vi "Global Resources Mod.vi"(7 "Path to All Nodes Resources":string="IONode\\Controls\\All Nodes Resources.ctl", 8 "error in":errorcluster, 10 "Number of SPI Devices on Bus":i32=1 min=1 step=1, 11 "Path to IO Node":path=path "D:/Documents/Projects/SPIAPI/IOEngineCode/Initialize Node Resources.vi") -> (0 "error out":errorcluster, 2 "Number of SPI Devices on Bus":i32=1 min=1 step=1, 3 "Path to IO Node":path=path "D:/Documents/Projects/SPIAPI/IOEngineCode/Initialize Node Resources.vi")   [LabVIEW 2014, in "Initialization and IO Node Scripting.lvlib"]
uses:
  Initialization and IO Node Scripting.lvlib
  <vilib>/Utility/traverseref.llb/TRef TravTarget.ctl
  <vilib>/Utility/traverseref.llb/VI Scripting - Traverse.lvlib
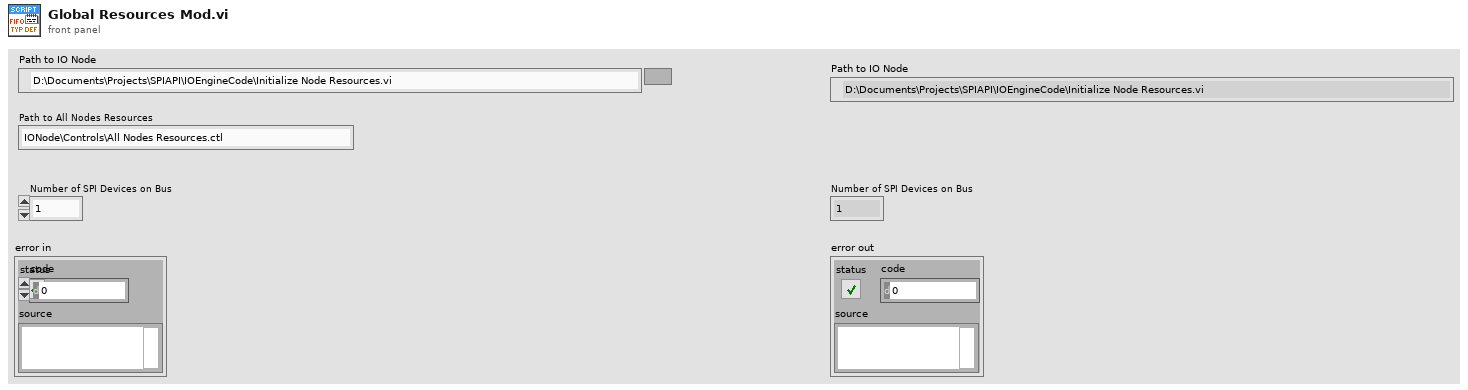
[diagram p1: front panel]
types:
  T1 = typedef "TRef TravTarget.ctl" = enum16{"FP", "BD", "Other"}
  T2 = typedef "LVPositionTypeDef.ctl" = cluster{"Left":i32, "Top":i32}
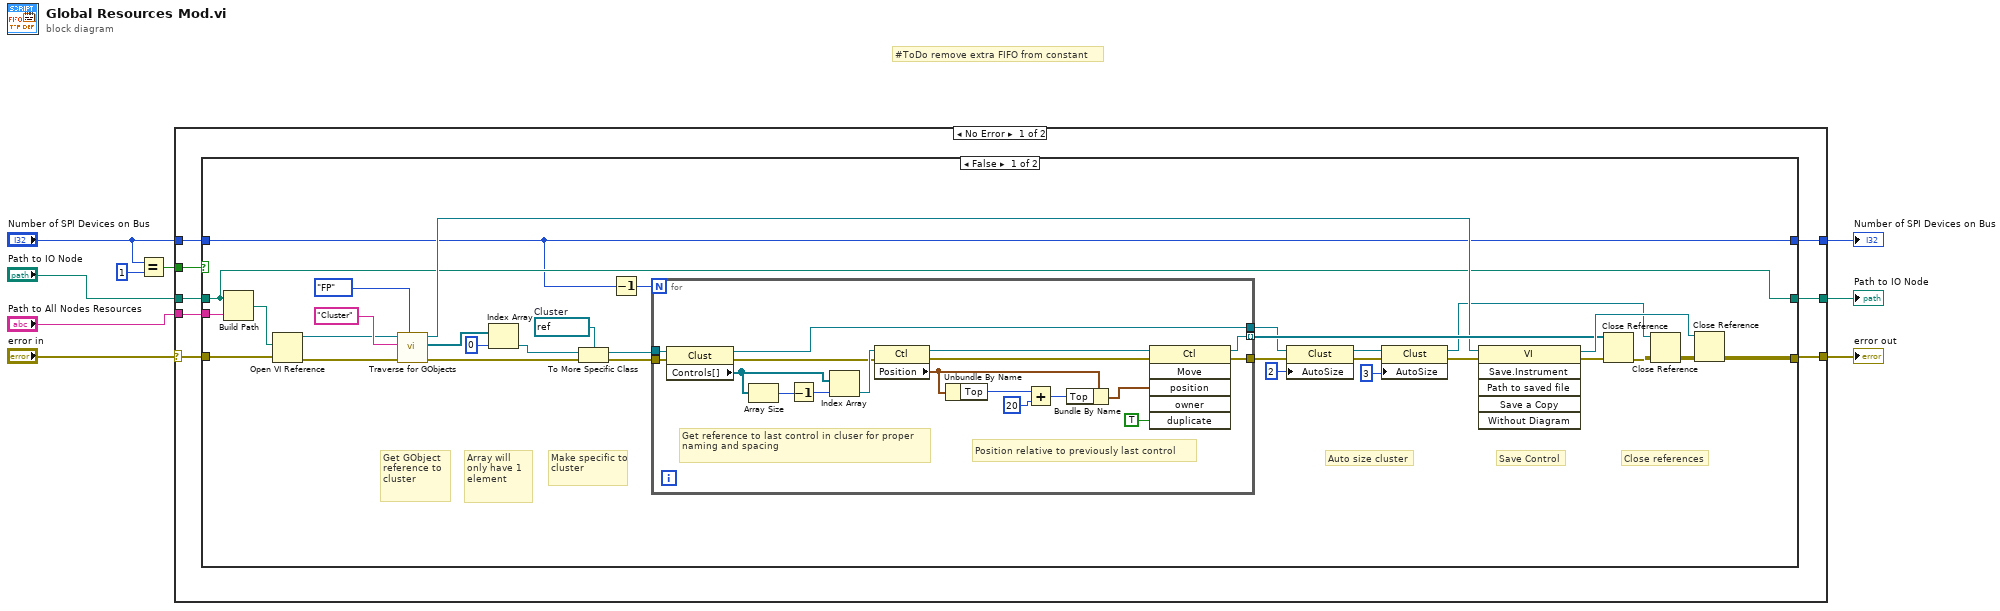
[diagram p0: block diagram]
diagram:
  # "#ToDo remove extra FIFO from constant"
  n1 = Equal?(x="Number of SPI Devices on Bus", y=1) -> (x = y?=w7:bool)
  n2 = case shown="No Error" "error in" {
    selector: "error in" -> [w13 w73]
    tunnel: [w17 w73] -> w9
    tunnel: "Path to IO Node" -> [w16 w71]
    tunnel: w7 -> [w15 _]
    tunnel: "Number of SPI Devices on Bus" -> [w14 w72]
    tunnel: [w11 w72] -> w3
    tunnel: [w12 w71] -> w2
    tunnel: "Path to All Nodes Resources" -> [w10 _]
    frame No Error {
      n3 = case shown="False" w15 {
        tunnel: [w48 w70] -> w17
        tunnel: w13 -> [w47 w70]
        tunnel: w16 -> [w28 w69]
        tunnel: w14 -> [w27 w68]
        tunnel: [w28 w69] -> w12
        tunnel: [w27 w68] -> w11
        tunnel: w10 -> [w26 _]
        frame False {
          w38 = refnum<vi> refnum  # Cluster
          # "Auto size cluster"
          # "Save Control"
          # "Close references"
          # "Array will only have 1 element"
          # "Make specific to cluster"
          # "Get GObject reference to cluster"
          n4 = Build Path(base path=w28, name or relative path=w26) -> (appended path=w46:path)
          n5 = Open VI Reference(vi path=w46, error in (no error)=w47) -> (vi reference=w43:refnum<vi>, error out=w37:errorcluster)  [unwired: 4 in]
          n6 = call <vilib>:"Traverse for GObjects.vi"("Traverse Target"=TRef_TravTarget."FP", "error in (no error)"=w37, "Class Name"="Cluster", "VI Refnum"=w43) -> ("error out"=w36:errorcluster, "References"=w42:refnum<vi>[], "dup VI Refnum"=w33:refnum<vi>)  [unwired: 4 in, 1 out]
          n7 = Index Array(array=w42, index=0) -> (element=w40:refnum<vi>)
          n8 = To More Specific Class(target class=w38, reference=w40, error in=w36) -> (specific class reference=w39:refnum<vi>, error out=w35:errorcluster)
          n9 = Decrement(x=w27) -> (x-1=w31:i32)
          n10 = for {
            N: w31 -> [_]
            tunnel: [w54] -> w20
            tunnel: w39 -> [w53]
            tunnel: w35 -> [w52]
            tunnel: [w51] -> w34 mode=indexing
            tunnel: [w50] -> w25
            # "Position relative to previously last control"
            # "Get reference to last control in cluser for proper naming and spacing"
            n11 = property class="Clust"(reference=w53, error in=w52) -> (reference out=w50:refnum<vi>, error out=w58:errorcluster, "Controls[]"=w57:refnum<vi>[])
            n12 = Array Size(array=w57) -> (size(s)=w67:i32)
            n13 = Decrement(x=w67) -> (x-1=w56:i32)
            n14 = Index Array(array=w57, index=w56) -> (element=w63:refnum<vi>)
            n15 = property class="Ctl"(reference=w63, error in=w58) -> (reference out=w64:refnum<vi>, error out=w65:errorcluster, "Position"=w61:T2)
            n16 = Unbundle By Name(w61) -> ("Top"=w60:i32)
            n17 = Add(x=w60, y=20) -> (x+y=w59:i32)
            n18 = Bundle By Name(cluster=w61, "Top"=w59) -> (w62:T2)
            n19 = invoke class="Ctl" method="Move"(reference=w64, error in=w65, "position"=w62, "duplicate"=TRUE ("Duplicate? (F)")) -> (reference out=w51:refnum<vi>, error out=w54:errorcluster)  [unwired: 2 in, 4 out]
          }
          n20 = property class="Clust"(reference=w25, error in=w20, "AutoSize"=u32 2 ("Auto Sizing")) -> (reference out=w23:refnum<vi>, error out=w22:errorcluster)
          n21 = property class="Clust"(reference=w23, error in=w22, "AutoSize"=u32 3 ("Auto Sizing")) -> (reference out=w18:refnum<vi>, error out=w19:errorcluster)
          n22 = invoke class="VI" method="Save.Instrument"(reference=w33, error in=w19) -> (reference out=w49:refnum<vi>, error out=w29:errorcluster)  [unwired: 4 in, 4 out]
          n23 = Close Reference(reference=w34, error in (no error)=w29) -> (error out=w30:errorcluster)
          n24 = Close Reference(reference=w18, error in (no error)=w30) -> (error out=w32:errorcluster)
          n25 = Close Reference(reference=w49, error in (no error)=w32) -> (error out=w48:errorcluster)
        }
        frame True {
        }
      }
    }
    frame Error {
    }
  }
  "error out" <- w9
  "Path to IO Node" <- w2
  "Number of SPI Devices on Bus" <- w3
